vi "test doublepush move.vi"() -> ()   [LabVIEW 2015]
uses:
  Chesslib/Position/Position.lvclass
  Chesslib/typedef/Piece.ctl
  Chesslib/typedef/Color.ctl
  Chesslib/typedef/Piece type.ctl
  Chesslib/typedef/Square.ctl
  Chesslib/typedef/File.ctl
  Chesslib/typedef/Rank.ctl
  Chesslib/Position/Position.lvclass/Position.ctl
  Chesslib/Chesslib.lvlib
  Chesslib/Moves/DoublePush/DoublePush.lvclass
  Chesslib/Board/Board.lvclass
panel:
  out "Board layout":cluster{"Occupied":bool, "Piece":T1}[][](array[cluster])
  out "Position out":refnum<class "Position.lvclass">
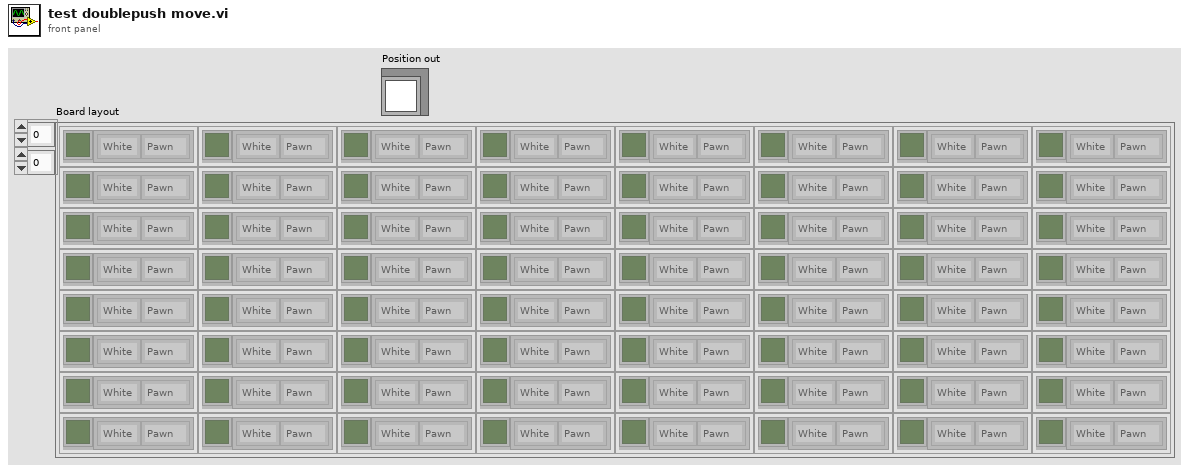
[diagram p1: front panel]
types:
  T1 = typedef "Chesslib.lvlib/Piece.ctl" = cluster{"Color":T2, "Type":T3}
  T2 = typedef "Chesslib.lvlib/Color.ctl" = enum16{"White", "Black"}
  T3 = typedef "Chesslib.lvlib/Piece type.ctl" = enum16{"Pawn", "Bishop", "Knight", "Rook", "Queen", "King"}
  T4 = typedef "Chesslib.lvlib/Square.ctl" = cluster{"File":T5, "Rank":T6}
  T5 = typedef "Chesslib.lvlib/File.ctl" = enum8{"a", "b", "c", "d", "e", "f", "g", "h"}
  T6 = typedef "Chesslib.lvlib/Rank.ctl" = enum8{"1", "2", "3", "4", "5", "6", "7", "8"}
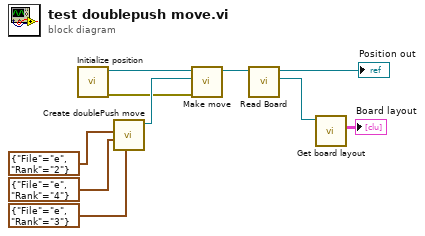
[diagram p0: block diagram]
diagram:
  n1 = call "Initialize position.vi"() -> ("error out"=w4:errorcluster, "Position out"=w10:refnum<class "Position.lvclass">)  [unwired: 10 in]
  n2 = call "Create doublePush move.vi"("enPassant target"=T4 {"File"=enum."e", "Rank"=enum."3"}, "Destination"=T4 {"File"=enum."e", "Rank"=enum."4"}, "Source"=T4 {"File"=enum."e", "Rank"=enum."2"}) -> ("DoublePush out"=w8:refnum<class "DoublePush.lvclass">)  [unwired: 8 in]
  n3 = call "Make move.vi"("error in (no error)"=w4, "Move"=w8, "Position in"=w10) -> ("Position out"=w9:refnum<class "Position.lvclass">)  [unwired: 7 in, 1 out]
  n4 = call "Read Board.vi"("Position in"=w9) -> ("Chesslib.lvlib:Board.lvclass"=w2:refnum<class "Board.lvclass">, "Position out"=→"Position out":refnum<class "Position.lvclass">)  [unwired: 9 in]
  n5 = call "Get board layout.vi"("Board in"=w2) -> ("Board layout"=→"Board layout":cluster{"Occupied":bool, "Piece":T1}[][])  [unwired: 9 in, 1 out]
